vi "WriteToDS.vi"(3 "Num Of Times To Send Message":u32, 4 "String To Send":string, 5 "DataSocket Refnum":refnum<k13>) -> (0 "error out":errorcluster)   [LabVIEW 2011]
doc: "This example illustrates using datasocket for writing out a waveform \n \nIt works for writing the data to local files, or to the DataSocket Server (for live data). \n \nTo use it with live data, start the DataSocket Server from the Start menu and run the DS Reader example with the dstp URL (dstp://localhost/wave, for example). Then select the same URL in this example and start this VI.\n \nThe Writer, Server, and Reader can all be on the same machine or different machines. The Writer's and Reader's URL should point to the machine that the DataSocket Server is on."
panel:
  out "String Sent":string
  out "Status":string
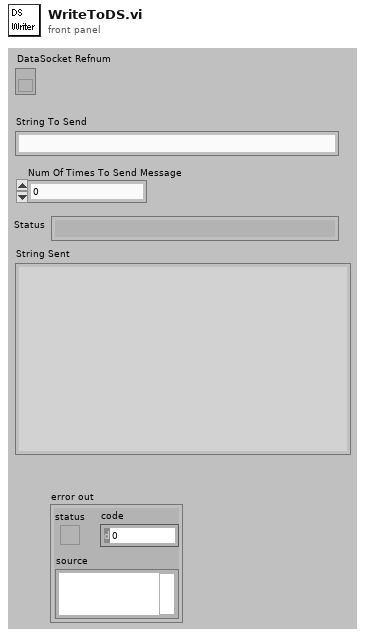
[diagram p1: front panel]
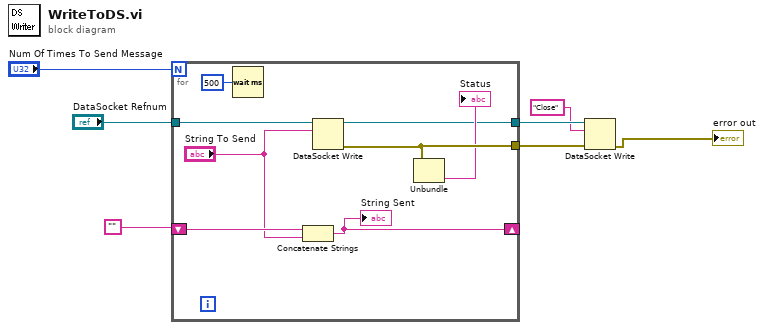
[diagram p0: block diagram]
diagram:
  n1 = for {
    N: "Num Of Times To Send Message" -> [_]
    tunnel: [w13] -> w3
    tunnel: "DataSocket Refnum" -> [w15]
    shift-right: [w10] -> _
    shift-left: "" -> [w11]
    tunnel: [w8] -> w4
    n2 = Wait (ms)(milliseconds to wait=u32 500) -> ()  [unwired: 1 out]
    n3 = Concatenate Strings(w11, "String To Send") -> (w10:string)
    "String Sent" <- w10
    n4 = DataSocket Write(10:"String To Send", 11:w15) -> (0:w13:errorcluster, 3:w8:refnum<k13>)  [unwired: 1 in, 2 out]
    n5 = Unbundle(w13) -> ("source"=→"Status":string)  [unwired: 2 out]
  }
  n6 = DataSocket Write(8:w3, 10:"Close", 11:w4) -> (0:→"error out":errorcluster)  [unwired: 3 out]
